vi "Example 4 - Value As.vi"() -> ()   [LabVIEW 2021]
uses:
  Omni-Bus/Omni_Bus.lvclass
  Omni-Bus/Support/Broad Types.ctl
  Local Bus/Local Bus.lvclass
  C:/Users/Tim/Documents/GitHub/Omni-Bus/Source/Omni-Bus/Bus Access/Bus_Access.lvclass
  <vilib>/Utility/Data Type/Type Definitions/Data Type.ctl
  Omni-Bus/Support/Read As/Read Numeric as DBL.vi
  Omni-Bus/Support/Read As/Read Value as String.vi
  Omni-Bus/Support/Read As/Read Value as Variant.vi
  <vilib>/TSA/Abstract Data Classes/Abs_Types/Numeric/Abs_Numeric.lvclass
  <vilib>/TSA/Abstract Data Classes/Abs_Types/Value/Abs_Value.lvclass
  Omni-Bus/Support/Write As/Write Variant as Value.vi
  Omni-Bus/Support/Write As/Write DBL as Numeric.vi
  Omni-Bus/Support/Write As/Write String as Value.vi
  <vilib>/Utility/Data Type/NI_Data Type.lvlib
panel:
  out "Variant":variant
  in  "Write Boolean as Variant Tag":string
  in  "Boolean":bool
  out "Write Boolean error":errorcluster
  in  "Write Value as String Tag":string
  in  "String":string
  out "Write String error":errorcluster
  out "Read Bool Error":errorcluster
  out "Read String error":errorcluster
  out "As String":string
  in  "Read Value as Variant Tag":string
  in  "Read Value as String Tag":string
  out "Read DBL error":errorcluster
  out "Write DBL error":errorcluster
  in  "Double":dbl
  in  "Write Numeric as DBL Tag":string
  in  "stop":bool
  out "Double":dbl format="%.2f"
  in  "Read Numeric as DBL Tag":string
  out "error out":errorcluster
  out "All Tags":string[](array[string])
  # "All Value Classes can be \nread and written as:\nVariant, \nString, (text)\nBinary String\nJSON String\n\nAll Numeric Types can be\nread and written to as another\nnumeric type and the classes\nlook after the casting."
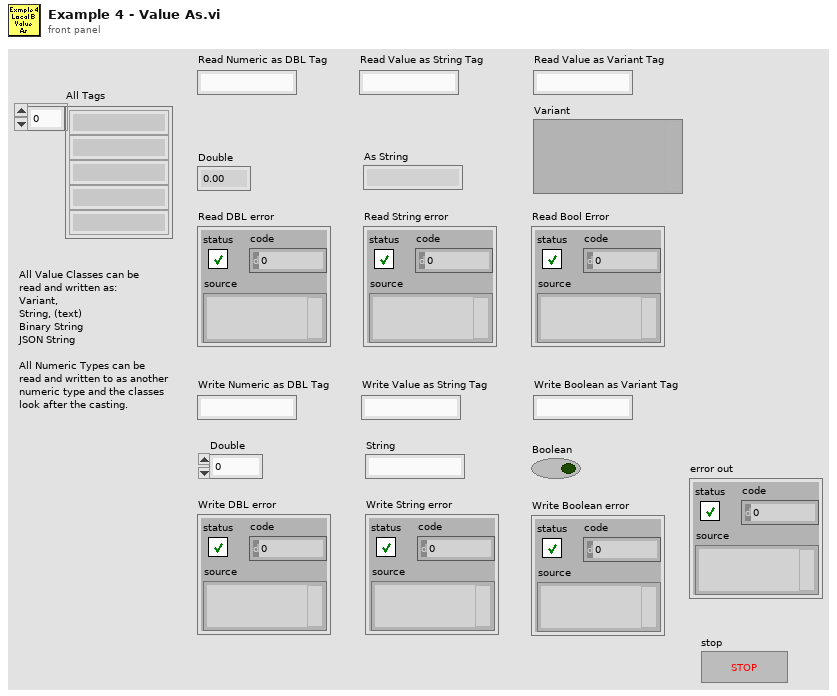
[diagram p1: front panel]
types:
  T1 = typedef "NI_Data Type.lvlib/Data Type.ctl" = enum8{"Invalid Type", "Void", "I8", "I16", "I32", "I64", "U8", "U16", "U32", "U64", "Single Float", "Double Float", "Extended Float", "Single Complex", "Double Complex", "Extended Complex", "Enum U8", "Enum U16", "Enum U32", "Enum U64", "Single Float With Unit", "Double Float With Unit", "Extended Float With Unit", "Single Complex with Unit", "Double Complex with Unit", "Extended Complex with Unit", "Boolean", "String", "Path", "Picture", "Tag", "Array", "Cluster", "Variant", "LV Variant", "Waveform", "Timestamp", "Digital Waveform", "Digital Data", "ExpressData", "Refnum", "External Data", "VI", "Poly VI", "LabVIEW Class Instance", "Fixed Point", "Set Collection", "Map Collection"}
  T2 = typedef "Omni_Bus.lvclass/Broad Types.ctl" = enum16{"All Tags", "NI Specific Type", "Boolean", "String", "Numeric", "Float", "Integer", "Collection", "All Value Types", "Non Value Types"}
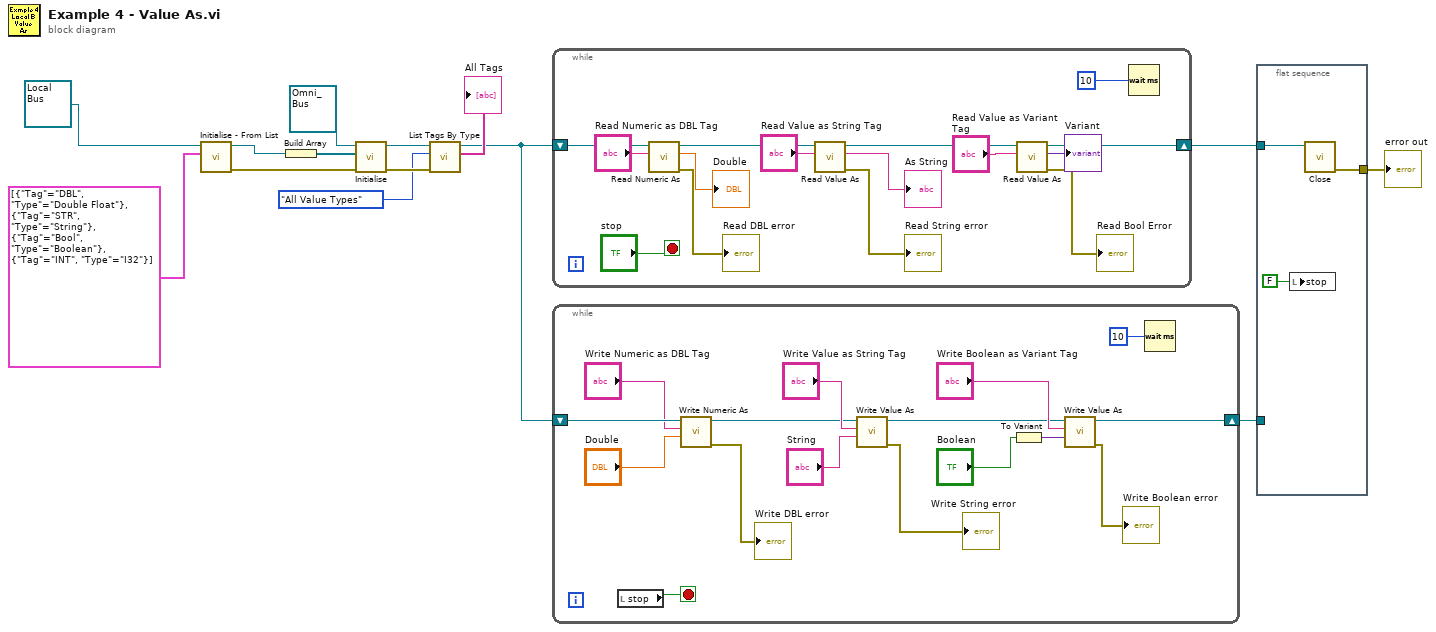
[diagram p0: block diagram]
diagram:
  n1 = call "Initialise - From List.vi"("Tag List"=cluster{"Tag":string, "Type":T1}[] [{"Tag"="DBL", "Type"=enum."Double Float"}, {"Tag"="STR", "Type"=enum."String"}, {"Tag"="Bool", "Type"=enum."Boolean"}, {"Tag"="INT", "Type"=enum."I32"}], "Local Bus in"=refnum<class "Local Bus.lvclass"> refnum ("Local Bus.lvclass")) -> ("error out"=w4:errorcluster, "Local Bus out"=w3:refnum<class "Local Bus.lvclass">)  [unwired: 8 in]
  n2 = Build Array(w3) -> (w13:refnum<class "Local Bus.lvclass">[])
  n3 = call-dynamic "Initialise.vi"("error in (no error)"=w4, "Bus Access"=w13, "Var Bus in"=refnum<class "Omni_Bus.lvclass"> refnum) -> ("error out"=w11:errorcluster, "Var Bus out"=w12:refnum<class "Omni_Bus.lvclass">)  [unwired: 7 in]
  n4 = call-dynamic "List Tags By Type.vi"("error in (no error)"=w11, "Broad Types"=Broad_Types."All Value Types", "Var Bus in"=w12) -> ("Tags"=→"All Tags":string[], "Var Bus out"=w6:refnum<class "Omni_Bus.lvclass">)  [unwired: 5 in, 2 out]
  n5 = while {
    shift-right: [w19] -> w7
    shift-left: w6 -> [w29]
    stop <- "stop" stop-if-true
    n6 = call-poly "Read Numeric As.vi"("Tag"="Read Numeric as DBL Tag", "Var Bus in"=w29) -> ("error out"=→"Read DBL error":errorcluster, "Numeric"=→"Double":dbl, "Var Bus out"=w22:refnum<class "Omni_Bus.lvclass">)  [unwired: 7 in]
    n7 = call-poly "Read Value As.vi"("Tag"="Read Value as String Tag", "Var Bus in"=w22) -> ("error out"=→"Read String error":errorcluster, "String"=→"As String":string, "Var Bus out"=w20:refnum<class "Omni_Bus.lvclass">)  [unwired: 7 in]
    n8 = call-poly "Read Value As.vi"("Tag"="Read Value as Variant Tag", "Var Bus in"=w20) -> ("error out"=→"Read Bool Error":errorcluster, "Variant"=→"Variant":variant, "Var Bus out"=w19:refnum<class "Omni_Bus.lvclass">)  [unwired: 7 in]
    n9 = Wait (ms)(milliseconds to wait=u32 10) -> ()  [unwired: 1 out]
  }
  n10 = while {
    shift-right: [w32] -> w5
    shift-left: w6 -> [w45]
    stop <- w42 stop-if-true
    n11 = local read "stop"() -> (w42:bool)
    n12 = call-poly "Write Numeric As.vi"("Numeric"="Double", "Tag"="Write Numeric as DBL Tag", "Omni_Bus in"=w45) -> ("error out"=→"Write DBL error":errorcluster, "Omni_Bus out"=w36:refnum<class "Omni_Bus.lvclass">)  [unwired: 7 in]
    n13 = call-poly "Write Value As.vi"("String"="String", "Tag"="Write Value as String Tag", "Var Bus in"=w36) -> ("error out"=→"Write String error":errorcluster, "Var Bus out"=w33:refnum<class "Omni_Bus.lvclass">)  [unwired: 7 in]
    n14 = To Variant(anything="Boolean") -> (Variant=w31:variant)
    n15 = call-poly "Write Value As.vi"("Variant"=w31, "Tag"="Write Boolean as Variant Tag", "Var Bus in"=w33) -> ("error out"=→"Write Boolean error":errorcluster, "Var Bus out"=w32:refnum<class "Omni_Bus.lvclass">)  [unwired: 7 in]
    n16 = Wait (ms)(milliseconds to wait=u32 10) -> ()  [unwired: 1 out]
  }
  n17 = flat-sequence {
    tunnel: [w48] -> w8
    tunnel: w7 -> [w47]
    tunnel: w5 -> [_]
    frame #0 {
      n18 = local write "stop"(FALSE ("stop")) -> ()
      n19 = call-dynamic "Close.vi"("Data in"=w47) -> ("error out"=w48:errorcluster)  [unwired: 9 in, 1 out]
    }
  }
  "error out" <- w8
